vi "getImage_action.vi"(0 "HGF_ImaqFg":refnum<class "HGF_ImaqFg.lvclass">, 2 "Image In":T1, 3 "Buffer Number":u32, 4 "Timeout (1000ms)":i32=1000, 5 "error in (no error)":errorcluster, 6 "Region of Interest":i32[](array[numeric]), 8 "Buffer Number Mode (Next)":T2) -> (11 "Frame Numbers":i32[](array[numeric]), 13 "Image Array":T1[](array[typedef]), 14 "dup HGF_ImaqFg":refnum<class "HGF_ImaqFg.lvclass">, 16 "Image Out":T1, 17 "Buffer Number Copied":i32, 18 "Buffer Index Copied":i32, 19 "error out":errorcluster)   [LabVIEW 2014, in "HGF_IMAQ.lvlib" / "HGF_ImaqFg.lvclass"]
doc: "Returns a copy of an acquired image. IMAQ Copy Acquired Buffer allows you to copy an image from onboard memory to system memory, or from driver-allocated system memory to user-allocated system memory.\n\nCall this VI only after calling IMAQdx Configure Acquisition.vi. If the image type does not match the video format of the camera, this VI changes the image type to a suitable format, at least for IMAQdx."
uses:
  HGF_ImaqFg.lvclass
  <vilib>/vision/driver/IMAQdx.llb/IMAQdx Buffer Number Mode.ctl
  <vilib>/vision/Image Controls.llb/IMAQ Image.ctl
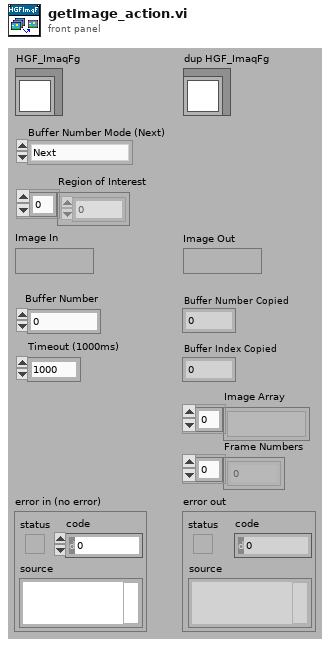
[diagram p1: front panel]
types:
  T1 = typedef "IMAQ Image.ctl" = refnum<image>
  T2 = typedef "NI_Vision_Acquisition_Software.lvlib/IMAQdx Buffer Number Mode.ctl" = enum32{"Next", "Last", "Buffer Number"}
  T3 = enum16{"Get Oldest", "Get Next Iteration", "Fail"}
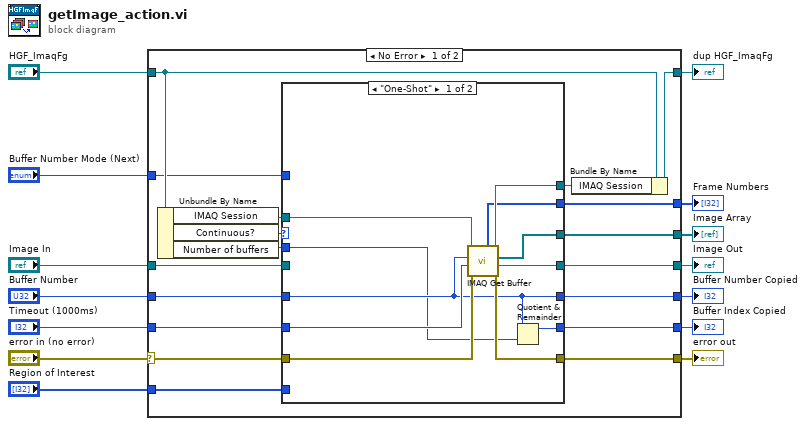
[diagram p0: block diagram]
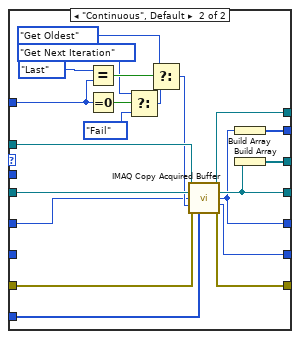
[diagram p2: hidden frame]
diagram:
  n1 = case shown="No Error" "error in (no error)" {
    selector: "error in (no error)" -> [w16 w65]
    tunnel: "Image In" -> [w32 w66]
    tunnel: [w31 w66] -> w13
    tunnel: "HGF_ImaqFg" -> [w29 w67]
    tunnel: [w27 w67] -> w11
    tunnel: "Buffer Number" -> [w26 _]
    tunnel: "Timeout (1000ms)" -> [w25 _]
    tunnel: [w24 _] -> w8
    tunnel: [w23 _] -> w7
    tunnel: [w22 w65] -> w6
    tunnel: "Region of Interest" -> [w21 _]
    tunnel: [w19 _] -> w4
    tunnel: [w17 _] -> w3
    tunnel: "Buffer Number Mode (Next)" -> [w15 _]
    frame No Error {
      n2 = Unbundle By Name(w29) -> ("IMAQ Session"=w30:refnum<k11>, "Continuous?"=w20:enum16{"One-Shot", "Continuous"}, "Number of buffers"=w18:u32)
      n3 = case shown="\"One-Shot\"" w20 {
        tunnel: w32 -> [_ w64]
        tunnel: [w40 w57] -> w31
        tunnel: w30 -> [w43 w63]
        tunnel: [w42 w62] -> w28
        tunnel: w26 -> [w35 w44]
        tunnel: w25 -> [w39 _]
        tunnel: w16 -> [w38 w61]
        tunnel: [w35 w54] -> w24
        tunnel: [w36 w60] -> w23
        tunnel: [w37 w59] -> w22
        tunnel: w21 -> [_ w58]
        tunnel: [w41 w56] -> w19
        tunnel: w18 -> [w34 _]
        tunnel: [w33 w55] -> w17
        tunnel: w15 -> [_ w47]
        frame "One-Shot" {
          n4 = call <vilib>:"IMAQ Get Buffer.vi"("error in (no error)"=w38, "Timeout (ms)"=w39, "Buffer Number (-1:all)"=w35, "IMAQ Session In"=w43) -> ("error out"=w37:errorcluster, "Image Out"=w40:T1, "Images Out"=w41:T1[], "IMAQ Session Out"=w42:refnum<k11>, "Frame Numbers"=w33:i32[])  [unwired: 3 out]
          n5 = Quotient & Remainder(x=w35, y=w34) -> (x-y*floor(x/y)=w36:u32)  [unwired: 1 out]
        }
        frame "Continuous", Default {
          n6 = Equal?(x=IMAQdx_Buffer_Number_Mode."Last" ("y"), y=w47) -> (x = y?=w50:bool)
          n7 = Equal To 0?(x=w47) -> (x = 0?=w53:bool)
          n8 = Select(t=T3."Get Next Iteration" ("Overwrite Mode"), s=w53, f=T3."Fail" ("Overwrite Mode")) -> (s? t:f=w49:T3)
          n9 = Select(t=T3."Get Oldest" ("Overwrite Mode"), s=w50, f=w49) -> (s? t:f=w48:T3)
          n10 = call <vilib>:"IMAQ Copy Acquired Buffer.vi"("IMAQ Session In"=w63, "Image In"=w64, "Buffer Number"=w44, "Overwrite Mode"=w48, "error in (no error)"=w61, "Region of Interest"=w58) -> ("IMAQ Session Out"=w62:refnum<k11>, "Image Out"=w57:T1, "Buffer Number Copied"=w54:i32, "Buffer Index Copied"=w60:i32, "error out"=w59:errorcluster)  [unwired: 5 out]
          n11 = Build Array(w54) -> (w55:i32[])
          n12 = Build Array(w57) -> (w56:T1[])
        }
      }
      n13 = Bundle By Name(cluster=w29, "IMAQ Session"=w28) -> (w27:refnum<class "HGF_ImaqFg.lvclass">)
    }
    frame Error {
    }
  }
  "error out" <- w6
  "dup HGF_ImaqFg" <- w11
  "Image Array" <- w4
  "Buffer Number Copied" <- w8
  "Buffer Index Copied" <- w7
  "Frame Numbers" <- w3
  "Image Out" <- w13
